vi "menuSelection.vi"(8 "error in (no error)":errorcluster, 9 "MenuRef":refnum<k9>, 10 "itemPath":string, 11 "ImageStreamViewer in":refnum<class "ImageStreamViewer.lvclass">) -> (0 "error out":errorcluster, 2 "close":bool, 3 "ImageStreamViewer out":refnum<class "ImageStreamViewer.lvclass">)   [LabVIEW 2009, in "Views.lvlib" / "Camera.lvlib" / "ImageStreamViewer.lvclass"]
uses:
  ImageStreamViewer.lvclass
  Tools/ImageProcessor/ImageAnalyser/AbsorptionAnalyser/AbsorptionAnalyser.lvclass
  Tools/ImageProcessor/ImageAnalyser/AbsorptionDS/AbsorptionDS.lvclass
  Tools/ImageProcessor/ImageAnalyser/FluorescenceAnalyser/FluorescenceAnalyser.lvclass
  Tools/ImageProcessor/ImageAnalyser/TemperatureAnalyser/TemperatureAnalyser.lvclass
  Tools/ImageProcessor/ImageAnalyser/FringeTesting/FringeTesting.lvclass
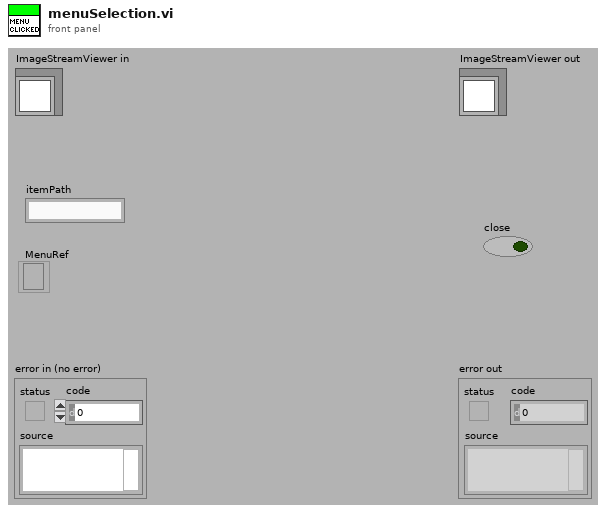
[diagram p1: front panel]
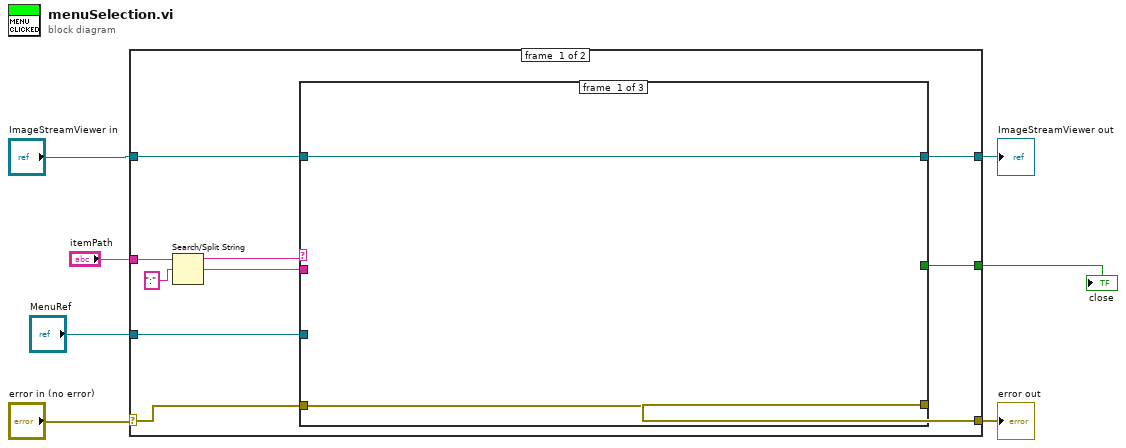
[diagram p0: block diagram]
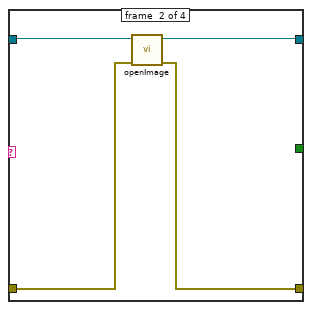
[diagram p3: hidden frame]
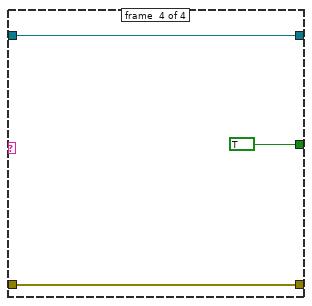
[diagram p5: hidden frame]
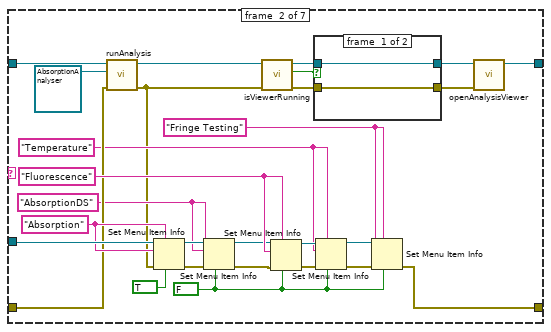
[diagram p7: hidden frame]
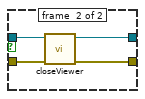
[diagram p8: hidden frame]
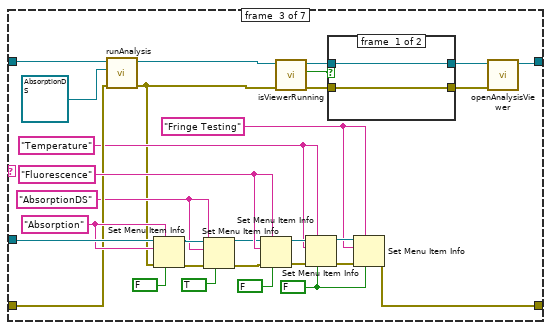
[diagram p9: hidden frame]
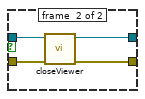
[diagram p10: hidden frame]
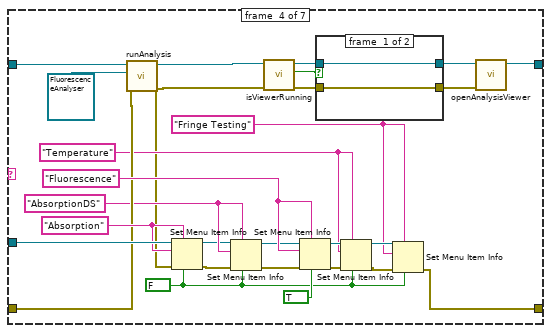
[diagram p11: hidden frame]
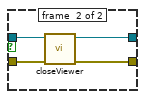
[diagram p12: hidden frame]
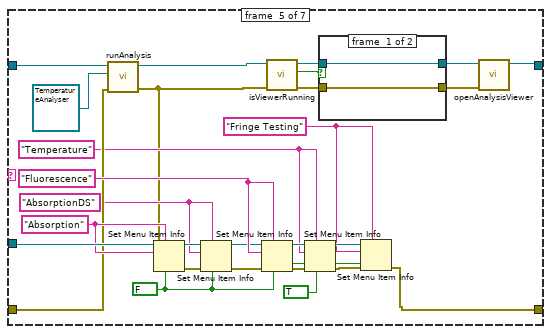
[diagram p13: hidden frame]
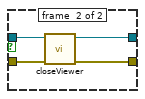
[diagram p14: hidden frame]
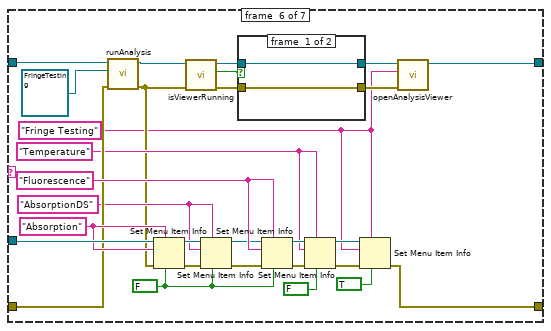
[diagram p15: hidden frame]
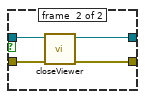
[diagram p16: hidden frame]
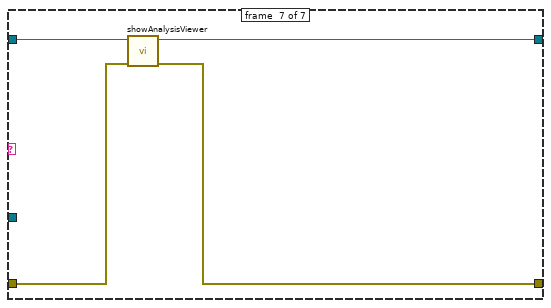
[diagram p17: hidden frame]
diagram:
  n1 = case shown="No Error" "error in (no error)" {
    selector: "error in (no error)" -> [w16 w223]
    tunnel: [w15 w223] -> w1
    tunnel: [w12 w222] -> w5
    tunnel: "ImageStreamViewer in" -> [w11 w222]
    tunnel: [w10 _] -> w6
    tunnel: "itemPath" -> [w9 _]
    tunnel: "MenuRef" -> [w8 _]
    frame #0 {
      n2 = Search/Split String(string=w9, search string/char (-)=":") -> (substring before match=w14:string, match + rest of string=w13:string)  [unwired: 1 in, 1 out]
      n3 = case shown="\"Analysis\"" w14 {
        tunnel: w16 -> [w18 w25 w39]
        tunnel: [w18 w24 w38] -> w15
        tunnel: w13 -> [_ w21 w40]
        tunnel: w11 -> [w19 w23 w42]
        tunnel: [w19 w22 w41] -> w12
        tunnel: [_ w20 _] -> w10
        tunnel: w8 -> [_ _ w37]
        frame #0 {
        }
        frame #1 {
          n4 = case shown="\":Close\"" w21 {
            tunnel: w25 -> [w26 w29 w32 w35]
            tunnel: [w26 w28 w32 w35] -> w24
            tunnel: w23 -> [w27 w31 w33 w36]
            tunnel: [w27 w30 w33 w36] -> w22
            tunnel: [_ _ _ TRUE] -> w20
            frame #0 {
            }
            frame #1 {
              n5 = call "openImage.vi"("error in (no error)"=w29, "ImageStreamViewer in"=w31) -> ("error out"=w28:errorcluster, "ImageStreamViewer out"=w30:refnum<class "ImageStreamViewer.lvclass">)  [unwired: 8 in]
            }
            frame #2 {
            }
            frame #3 {
            }
          }
        }
        frame #2 {
          n6 = case shown="\":Absorption\"" w40 {
            tunnel: w42 -> [w44 w68 w103 w139 w173 w208 w221]
            tunnel: [w44 w45 w79 w115 w149 w184 w220] -> w41
            tunnel: w39 -> [w43 w67 w102 w138 w172 w207 w219]
            tunnel: [w43 w53 w89 w125 w159 w193 w218] -> w38
            tunnel: w37 -> [_ w72 w108 w142 w176 w211 _]
            frame #0 {
            }
            frame #1 {
              w55 = "Fringe Testing"
              w58 = "AbsorptionDS"
              w63 = "Temperature"
              w70 = "Absorption"
              w69 = "Fluorescence"
              w54 = FALSE
              n7 = call "runAnalysis.vi"("error in (no error)"=w67, "ImageAnalyser"=refnum<class "AbsorptionAnalyser.lvclass"> refnum ("Tools.lvlib:Imaging.lvlib:AbsorptionAnalyser.lvclass"), "ImageStreamViewer in"=w68) -> ("error out"=w46:errorcluster, "ImageStreamViewer out"=w47:refnum<class "ImageStreamViewer.lvclass">)  [unwired: 7 in]
              n8 = Set Menu Item Info(6:TRUE, 7:w70, 8:w46, 10:w70, 11:w72) -> (0:w60:errorcluster, 3:w62:refnum<k9>)  [unwired: 2 in]
              n9 = Set Menu Item Info(6:w54, 7:w58, 8:w60, 10:w58, 11:w62) -> (0:w59:errorcluster, 3:w61:refnum<k9>)  [unwired: 2 in]
              n10 = call "isViewerRunning.vi"("error in (no error)"=w46, "ImageStreamViewer in"=w47) -> ("error out"=w51:errorcluster, "running?"=w50:bool, "ImageStreamViewer out"=w52:refnum<class "ImageStreamViewer.lvclass">)  [unwired: 7 in]
              n11 = Set Menu Item Info(6:w54, 7:w69, 8:w59, 10:w69, 11:w61) -> (0:w65:errorcluster, 3:w64:refnum<k9>)  [unwired: 2 in]
              n12 = case shown="True" w50 {
                tunnel: w52 -> [w74 w78]
                tunnel: w51 -> [w73 w77]
                tunnel: [w74 w76] -> w49
                tunnel: [w73 w75] -> w48
                frame #0 {
                }
                frame #1 {
                  n13 = call "closeViewer.vi"("error in (no error)"=w77, "ImageStreamViewer in"=w78) -> ("error out"=w75:errorcluster, "ImageStreamViewer out"=w76:refnum<class "ImageStreamViewer.lvclass">)  [unwired: 8 in]
                }
              }
              n14 = Set Menu Item Info(6:w54, 7:w63, 8:w65, 10:w63, 11:w64) -> (0:w56:errorcluster, 3:w57:refnum<k9>)  [unwired: 2 in]
              n15 = Set Menu Item Info(6:w54, 7:w55, 8:w56, 10:w55, 11:w57) -> (0:w53:errorcluster)  [unwired: 2 in, 1 out]
              n16 = call "openAnalysisViewer.vi"("error in (no error)"=w48, "ImageStreamViewer in"=w49) -> ("ImageStreamViewer out"=w45:refnum<class "ImageStreamViewer.lvclass">)  [unwired: 8 in, 1 out]
            }
            frame #2 {
              w87 = "Fringe Testing"
              w92 = "AbsorptionDS"
              w99 = "Temperature"
              w88 = FALSE
              w105 = "Absorption"
              w104 = "Fluorescence"
              n17 = call "runAnalysis.vi"("error in (no error)"=w102, "ImageAnalyser"=refnum<class "AbsorptionDS.lvclass"> refnum ("Tools.lvlib:Imaging.lvlib:AbsorptionDS.lvclass"), "ImageStreamViewer in"=w103) -> ("error out"=w80:errorcluster, "ImageStreamViewer out"=w81:refnum<class "ImageStreamViewer.lvclass">)  [unwired: 7 in]
              n18 = Set Menu Item Info(6:FALSE, 7:w105, 8:w80, 10:w105, 11:w108) -> (0:w95:errorcluster, 3:w96:refnum<k9>)  [unwired: 2 in]
              n19 = Set Menu Item Info(6:TRUE, 7:w92, 8:w95, 10:w92, 11:w96) -> (0:w94:errorcluster, 3:w97:refnum<k9>)  [unwired: 2 in]
              n20 = Set Menu Item Info(6:FALSE, 7:w104, 8:w94, 10:w104, 11:w97) -> (0:w101:errorcluster, 3:w100:refnum<k9>)  [unwired: 2 in]
              n21 = call "isViewerRunning.vi"("error in (no error)"=w80, "ImageStreamViewer in"=w81) -> ("error out"=w85:errorcluster, "running?"=w84:bool, "ImageStreamViewer out"=w86:refnum<class "ImageStreamViewer.lvclass">)  [unwired: 7 in]
              n22 = Set Menu Item Info(6:w88, 7:w99, 8:w101, 10:w99, 11:w100) -> (0:w90:errorcluster, 3:w91:refnum<k9>)  [unwired: 2 in]
              n23 = case shown="True" w84 {
                tunnel: w86 -> [w110 w114]
                tunnel: w85 -> [w109 w113]
                tunnel: [w110 w112] -> w83
                tunnel: [w109 w111] -> w82
                frame #0 {
                }
                frame #1 {
                  n24 = call "closeViewer.vi"("error in (no error)"=w113, "ImageStreamViewer in"=w114) -> ("error out"=w111:errorcluster, "ImageStreamViewer out"=w112:refnum<class "ImageStreamViewer.lvclass">)  [unwired: 8 in]
                }
              }
              n25 = Set Menu Item Info(6:w88, 7:w87, 8:w90, 10:w87, 11:w91) -> (0:w89:errorcluster)  [unwired: 2 in, 1 out]
              n26 = call "openAnalysisViewer.vi"("error in (no error)"=w82, "ImageStreamViewer in"=w83) -> ("ImageStreamViewer out"=w79:refnum<class "ImageStreamViewer.lvclass">)  [unwired: 8 in, 1 out]
            }
            frame #3 {
              w123 = "Fringe Testing"
              w133 = "AbsorptionDS"
              w134 = "Temperature"
              w141 = "Absorption"
              w140 = "Fluorescence"
              w124 = FALSE
              n27 = call "runAnalysis.vi"("error in (no error)"=w138, "ImageAnalyser"=refnum<class "FluorescenceAnalyser.lvclass"> refnum ("Tools.lvlib:Imaging.lvlib:FluorescenceAnalyser.lvclass"), "ImageStreamViewer in"=w139) -> ("error out"=w116:errorcluster, "ImageStreamViewer out"=w117:refnum<class "ImageStreamViewer.lvclass">)  [unwired: 7 in]
              n28 = Set Menu Item Info(6:w124, 7:w141, 8:w116, 10:w141, 11:w142) -> (0:w130:errorcluster, 3:w132:refnum<k9>)  [unwired: 2 in]
              n29 = Set Menu Item Info(6:w124, 7:w133, 8:w130, 10:w133, 11:w132) -> (0:w129:errorcluster, 3:w131:refnum<k9>)  [unwired: 2 in]
              n30 = call "isViewerRunning.vi"("error in (no error)"=w116, "ImageStreamViewer in"=w117) -> ("error out"=w121:errorcluster, "running?"=w120:bool, "ImageStreamViewer out"=w122:refnum<class "ImageStreamViewer.lvclass">)  [unwired: 7 in]
              n31 = Set Menu Item Info(6:TRUE, 7:w140, 8:w129, 10:w140, 11:w131) -> (0:w135:errorcluster, 3:w136:refnum<k9>)  [unwired: 2 in]
              n32 = case shown="True" w120 {
                tunnel: w122 -> [w144 w148]
                tunnel: w121 -> [w143 w147]
                tunnel: [w144 w146] -> w119
                tunnel: [w143 w145] -> w118
                frame #0 {
                }
                frame #1 {
                  n33 = call "closeViewer.vi"("error in (no error)"=w147, "ImageStreamViewer in"=w148) -> ("error out"=w145:errorcluster, "ImageStreamViewer out"=w146:refnum<class "ImageStreamViewer.lvclass">)  [unwired: 8 in]
                }
              }
              n34 = Set Menu Item Info(6:w124, 7:w134, 8:w135, 10:w134, 11:w136) -> (0:w126:errorcluster, 3:w127:refnum<k9>)  [unwired: 2 in]
              n35 = Set Menu Item Info(6:w124, 7:w123, 8:w126, 10:w123, 11:w127) -> (0:w125:errorcluster)  [unwired: 2 in, 1 out]
              n36 = call "openAnalysisViewer.vi"("error in (no error)"=w118, "ImageStreamViewer in"=w119) -> ("ImageStreamViewer out"=w115:refnum<class "ImageStreamViewer.lvclass">)  [unwired: 8 in, 1 out]
            }
            frame #4 {
              w157 = "Fringe Testing"
              w162 = "AbsorptionDS"
              w168 = "Temperature"
              w175 = "Absorption"
              w174 = "Fluorescence"
              w158 = FALSE
              n37 = call "runAnalysis.vi"("error in (no error)"=w172, "ImageAnalyser"=refnum<class "TemperatureAnalyser.lvclass"> refnum ("Tools.lvlib:Imaging.lvlib:TemperatureAnalyser.lvclass"), "ImageStreamViewer in"=w173) -> ("error out"=w150:errorcluster, "ImageStreamViewer out"=w151:refnum<class "ImageStreamViewer.lvclass">)  [unwired: 7 in]
              n38 = Set Menu Item Info(6:w158, 7:w175, 8:w150, 10:w175, 11:w176) -> (0:w164:errorcluster, 3:w166:refnum<k9>)  [unwired: 2 in]
              n39 = Set Menu Item Info(6:w158, 7:w162, 8:w164, 10:w162, 11:w166) -> (0:w163:errorcluster, 3:w165:refnum<k9>)  [unwired: 2 in]
              n40 = Set Menu Item Info(6:w158, 7:w174, 8:w163, 10:w174, 11:w165) -> (0:w170:errorcluster, 3:w169:refnum<k9>)  [unwired: 2 in]
              n41 = call "isViewerRunning.vi"("error in (no error)"=w150, "ImageStreamViewer in"=w151) -> ("error out"=w155:errorcluster, "running?"=w154:bool, "ImageStreamViewer out"=w156:refnum<class "ImageStreamViewer.lvclass">)  [unwired: 7 in]
              n42 = Set Menu Item Info(6:TRUE, 7:w168, 8:w170, 10:w168, 11:w169) -> (0:w160:errorcluster, 3:w161:refnum<k9>)  [unwired: 2 in]
              n43 = case shown="True" w154 {
                tunnel: w156 -> [w178 w182]
                tunnel: w155 -> [w177 w181]
                tunnel: [w178 w180] -> w153
                tunnel: [w177 w179] -> w152
                frame #0 {
                }
                frame #1 {
                  n44 = call "closeViewer.vi"("error in (no error)"=w181, "ImageStreamViewer in"=w182) -> ("error out"=w179:errorcluster, "ImageStreamViewer out"=w180:refnum<class "ImageStreamViewer.lvclass">)  [unwired: 8 in]
                }
              }
              n45 = Set Menu Item Info(6:w158, 7:w157, 8:w160, 10:w157, 11:w161) -> (0:w159:errorcluster)  [unwired: 2 in, 1 out]
              n46 = call "openAnalysisViewer.vi"("error in (no error)"=w152, "ImageStreamViewer in"=w153) -> ("ImageStreamViewer out"=w149:refnum<class "ImageStreamViewer.lvclass">)  [unwired: 8 in, 1 out]
            }
            frame #5 {
              w183 = "Fringe Testing"
              w197 = "AbsorptionDS"
              w204 = "Temperature"
              w210 = "Absorption"
              w209 = "Fluorescence"
              w198 = FALSE
              n47 = call "runAnalysis.vi"("error in (no error)"=w207, "ImageAnalyser"=refnum<class "FringeTesting.lvclass"> refnum ("Tools.lvlib:Imaging.lvlib:FringeTesting.lvclass"), "ImageStreamViewer in"=w208) -> ("error out"=w190:errorcluster, "ImageStreamViewer out"=w191:refnum<class "ImageStreamViewer.lvclass">)  [unwired: 7 in]
              n48 = Set Menu Item Info(6:w198, 7:w210, 8:w190, 10:w210, 11:w211) -> (0:w200:errorcluster, 3:w202:refnum<k9>)  [unwired: 2 in]
              n49 = call "isViewerRunning.vi"("error in (no error)"=w190, "ImageStreamViewer in"=w191) -> ("error out"=w188:errorcluster, "running?"=w187:bool, "ImageStreamViewer out"=w189:refnum<class "ImageStreamViewer.lvclass">)  [unwired: 7 in]
              n50 = Set Menu Item Info(6:w198, 7:w197, 8:w200, 10:w197, 11:w202) -> (0:w199:errorcluster, 3:w201:refnum<k9>)  [unwired: 2 in]
              n51 = case shown="True" w187 {
                tunnel: w189 -> [w213 w217]
                tunnel: w188 -> [w212 w216]
                tunnel: [w213 w215] -> w186
                tunnel: [w212 w214] -> w185
                frame #0 {
                }
                frame #1 {
                  n52 = call "closeViewer.vi"("error in (no error)"=w216, "ImageStreamViewer in"=w217) -> ("error out"=w214:errorcluster, "ImageStreamViewer out"=w215:refnum<class "ImageStreamViewer.lvclass">)  [unwired: 8 in]
                }
              }
              n53 = Set Menu Item Info(6:w198, 7:w209, 8:w199, 10:w209, 11:w201) -> (0:w206:errorcluster, 3:w205:refnum<k9>)  [unwired: 2 in]
              n54 = Set Menu Item Info(6:FALSE, 7:w204, 8:w206, 10:w204, 11:w205) -> (0:w195:errorcluster, 3:w196:refnum<k9>)  [unwired: 2 in]
              n55 = Set Menu Item Info(6:TRUE, 7:w183, 8:w195, 10:w183, 11:w196) -> (0:w193:errorcluster)  [unwired: 2 in, 1 out]
              n56 = call "openAnalysisViewer.vi"("error in (no error)"=w185, "whichViewer"=w183, "ImageStreamViewer in"=w186) -> ("ImageStreamViewer out"=w184:refnum<class "ImageStreamViewer.lvclass">)  [unwired: 7 in, 1 out]
            }
            frame #6 {
              n57 = call "showAnalysisViewer.vi"("error in (no error)"=w219, "ImageStreamViewer in"=w221) -> ("error out"=w218:errorcluster, "ImageStreamViewer out"=w220:refnum<class "ImageStreamViewer.lvclass">)  [unwired: 8 in]
            }
          }
        }
      }
    }
    frame #1 {
    }
  }
  "error out" <- w1
  "ImageStreamViewer out" <- w5
  "close" <- w6
